vi "StartAsyncCall.vi"(11 "Actor":refnum<class "Actor.lvclass">) -> (0 "Error":errorcluster, 3 "PreSetup":T1)   [LabVIEW 2020, in "jettl.lvlib"]
uses:
  jettl.lvlib
  AsyncCall.vi
  PreSetup.ctl
  Actor/Actor.lvclass
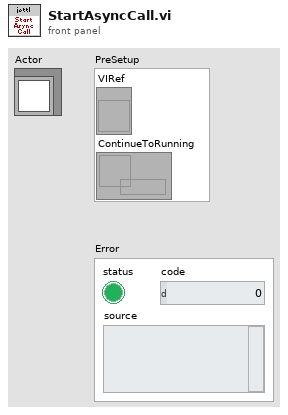
[diagram p1: front panel]
types:
  T1 = typedef "jettl.lvlib/PreSetup.ctl" = cluster{"VIRef":refnum<vi>, "ContinueToRunning":refnum<queue>}
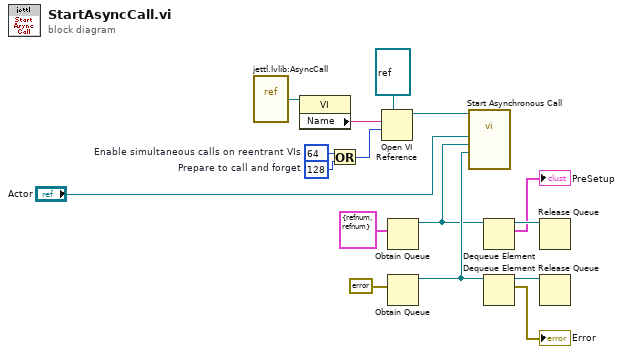
[diagram p0: block diagram]
diagram:
  w6 = 64  # Enable simultaneous calls on reentrant VIs
  w7 = 128  # Prepare to call and forget
  n1 = vi-ref "jettl.lvlib:AsyncCall.vi"() -> (w9:refnum<vi>)
  n2 = property class="VI"(reference=w9) -> ("Name"=w10:string)  [unwired: 1 in, 2 out]
  n3 = Or(x=w6, y=w7) -> (x .or. y?=w5:i32)
  n4 = Open VI Reference(type specifier VI Refnum (for type only)=refnum<vi> refnum, vi path=w10, options=w5) -> (vi reference=w4:refnum<vi>)  [unwired: 3 in, 1 out]
  n5 = Obtain Queue(element data type=T1 {"VIRef"=refnum, "ContinueToRunning"=refnum} ("PreSetup")) -> (queue out=w3:refnum<queue>)  [unwired: 4 in, 2 out]
  n6 = Obtain Queue(element data type=errorcluster {"status"=FALSE, "code"=0, "source"=""} ("Error")) -> (queue out=w14:refnum<queue>)  [unwired: 4 in, 2 out]
  n7 = call-by-ref "Start Asynchronous Call"(reference=w4, "ErrorQueue"=w14, "PreSetupQueue"=w3, "Actor"="Actor") -> ()  [unwired: 10 in, 2 out]
  n8 = Dequeue Element(queue=w3) -> (queue out=w2:refnum<queue>, element=→"PreSetup":T1)  [unwired: 2 in, 2 out]
  n9 = Dequeue Element(queue=w14) -> (queue out=w12:refnum<queue>, element=→"Error":errorcluster)  [unwired: 2 in, 2 out]
  n10 = Release Queue(queue=w2) -> ()  [unwired: 2 in, 3 out]
  n11 = Release Queue(queue=w12) -> ()  [unwired: 2 in, 3 out]
